vi "Init File.vi"(7 "create file if necessary (T)":bool=TRUE, 8 "error in (no error)":errorcluster, 10 "configuration file path":path, 11 "Parameter INI File in":refnum<class "Parameter INI File.lvclass">) -> (0 "error out":errorcluster, 3 "Parameter INI File out":refnum<class "Parameter INI File.lvclass">)   [LabVIEW 2019, in "CD Parameter Manager API.lvlib" / "Parameter INI File.lvclass"]
uses:
  Parameter INI File.lvclass
  C:/Repositories/UI-Control-Initializer-API/Source/Parameter Generic File/Parameter Generic File.lvclass
  Parameter Generic File/Parameter Generic File.lvclass/Parameter Generic File.ctl
  Parameter INI File.lvclass/Parameter INI File.ctl
  Parameter Generic File/Member Accessors/Read File Path.vi
  <vilib>/Utility/config.llb/NI_LVConfig.lvlib
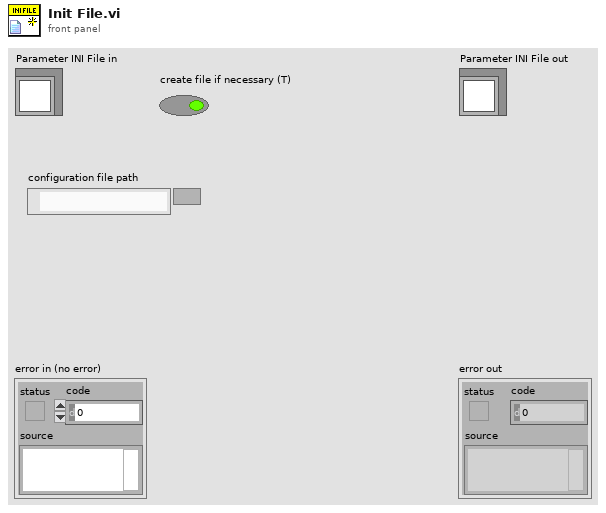
[diagram p1: front panel]
types:
  T1 = typedef "NI_LVConfig.lvlib/Config Data RefNum.ctl" = refnum<k1>
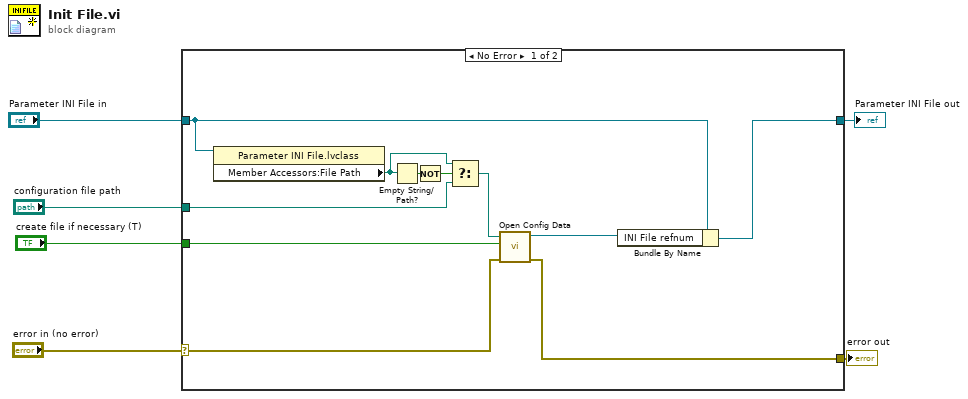
[diagram p0: block diagram]
diagram:
  n1 = case shown="No Error" "error in (no error)" {
    selector: "error in (no error)" -> [w14 w18]
    tunnel: [w17 w19] -> w5
    tunnel: "Parameter INI File in" -> [w7 w19]
    tunnel: "configuration file path" -> [w10 _]
    tunnel: "create file if necessary (T)" -> [w15 _]
    tunnel: [w13 w18] -> w1
    frame No Error {
      n2 = property class="Parameter INI File.lvclass"(reference=w7) -> ("Member Accessors:File Path"=w9:path)  [unwired: 1 in, 2 out]
      n3 = Empty String/Path?(string/path=w9) -> (empty?=w12:bool)
      n4 = Not(x=w12) -> (.not. x?=w11:bool)
      n5 = Select(t=w9, s=w11, f=w10) -> (s? t:f=w8:path)
      n6 = call <vilib>:"Open Config Data.vi"("error in (no error)"=w14, "create file if necessary (T)"=w15, "configuration file path"=w8) -> ("error out"=w13:errorcluster, "refnum"=w16:T1)  [unwired: 6 in, 1 out]
      n7 = Bundle By Name(cluster=w7, "INI File refnum"=w16) -> (w17:refnum<class "Parameter INI File.lvclass">)
    }
    frame Error {
    }
  }
  "error out" <- w1
  "Parameter INI File out" <- w5
